vi "FindMW (SubVI).vi"(7 "OptionPACK5":T1={"MagicWordStr"="xV4\u0012", "Header size"=56, "Проверка CRC8"=TRUE, "Проверка конца пакета"=FALSE, "GainCompens"=FALSE, "Неотбрасывать BadEnd пакеты"=TRUE, "Неотбрасывать BadCRC пакеты"=TRUE, "Привести к 1"=FALSE, "GainCoef"=FALSE, "K_scale"=0.0, "ScaleOrdinate"=enum."Проценты"}, 8 "error in":errorcluster, 11 "string in":string="xV4\u0012\u0002\u0000\u0000\u0000pМC\u0016њwѕa\u0000\u0010\u0000‹\u0000\u0000\u0000\u0000\u0000\u0000\u0000\u0000\u0000\u0000\u0000\u0000\u0000\u0000\u0000\u0000\u0000\u0000\u0000\u0000o\u0012ѓ9\u0000\u0000\u0000\u0000\u0000\u0000\u0000\u0000+\u0019\u0000\u0000\u00002”И\u0000z\u0011") -> (0 "error out":errorcluster, 1 "MWFind":bool, 2 "offset":i32=4)   [LabVIEW 2017]
uses:
  Control_EU/OptionPACK5.ctl
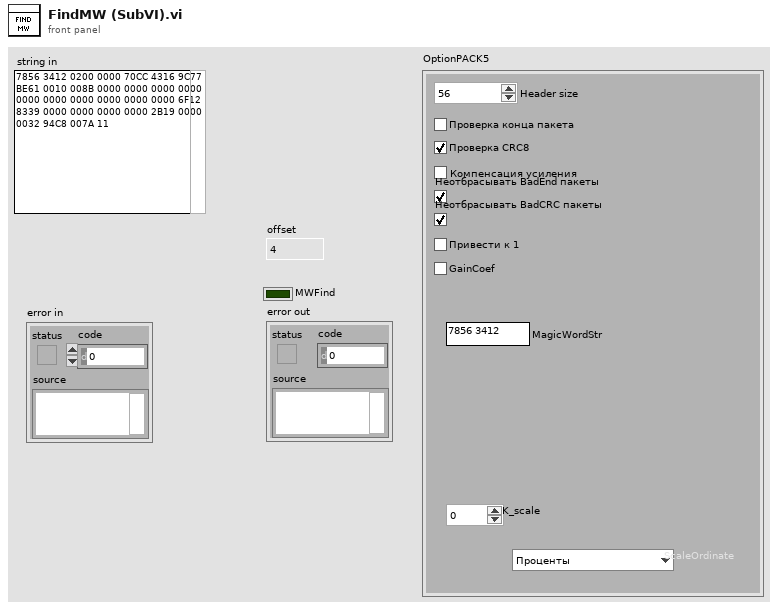
[diagram p1: front panel]
types:
  T1 = typedef "OptionPACK5.ctl" = cluster{"MagicWordStr":string, "Header size":u32, "Проверка CRC8":bool, "Проверка конца пакета":bool, "GainCompens":bool, "Неотбрасывать BadEnd пакеты":bool, "Неотбрасывать BadCRC пакеты":bool, "Привести к 1":bool, "GainCoef":bool, "K_scale":dbl, "ScaleOrdinate":enum16{"Отсчеты АЦП (±32767)", "Проценты", "Вольты", "дБмкВ (отн. 1 мкВ)", "Отсчеты АЦП (±1)"}}
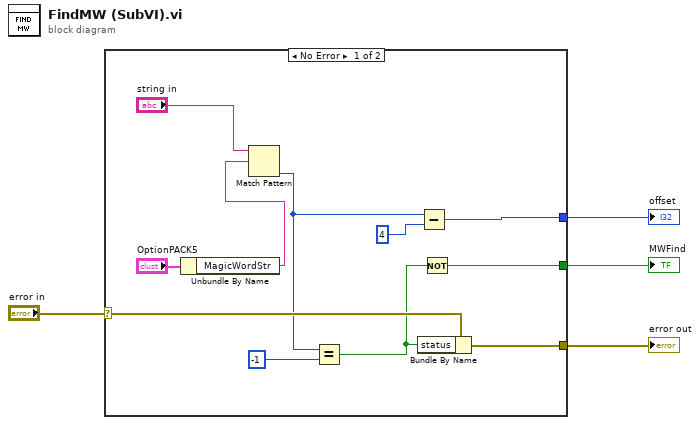
[diagram p0: block diagram]
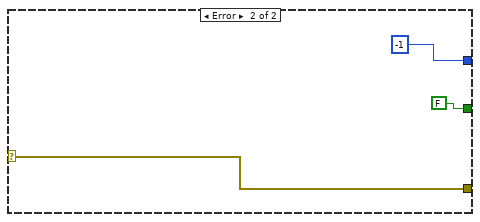
[diagram p2: hidden frame]
diagram:
  n1 = case shown="No Error" "error in" {
    selector: "error in" -> [w15 w18]
    tunnel: [w13 w18] -> w3
    tunnel: [w8 -1 ("offset past match")] -> w1
    tunnel: [w11 FALSE] -> w2
    frame No Error {
      n2 = Unbundle By Name("OptionPACK5") -> ("MagicWordStr"=w5:string)
      n3 = Match Pattern(string="string in", regular expression=w5) -> (offset past match=w10:i32)  [unwired: 1 in, 3 out]
      n4 = Equal?(x=w10, y=-1) -> (x = y?=w12:bool)
      n5 = Bundle By Name(cluster=w15, "status"=w12) -> (w13:errorcluster)
      n6 = Subtract(x=w10, y=4) -> (x-y=w8:i32)
      n7 = Not(x=w12) -> (.not. x?=w11:bool)
    }
    frame Error {
    }
  }
  "error out" <- w3
  "offset" <- w1
  "MWFind" <- w2
